vi "Template Rename.vi"(6 "ROI":string, 7 "Root Path":path, 8 "error in (no error)":errorcluster, 9 "Project List Idx":u16, 10 "Project List":string[](array[string])) -> (0 "error out":errorcluster)   [LabVIEW 2019]
uses:
  ROI/Controls/ROI_List_Action.ctl
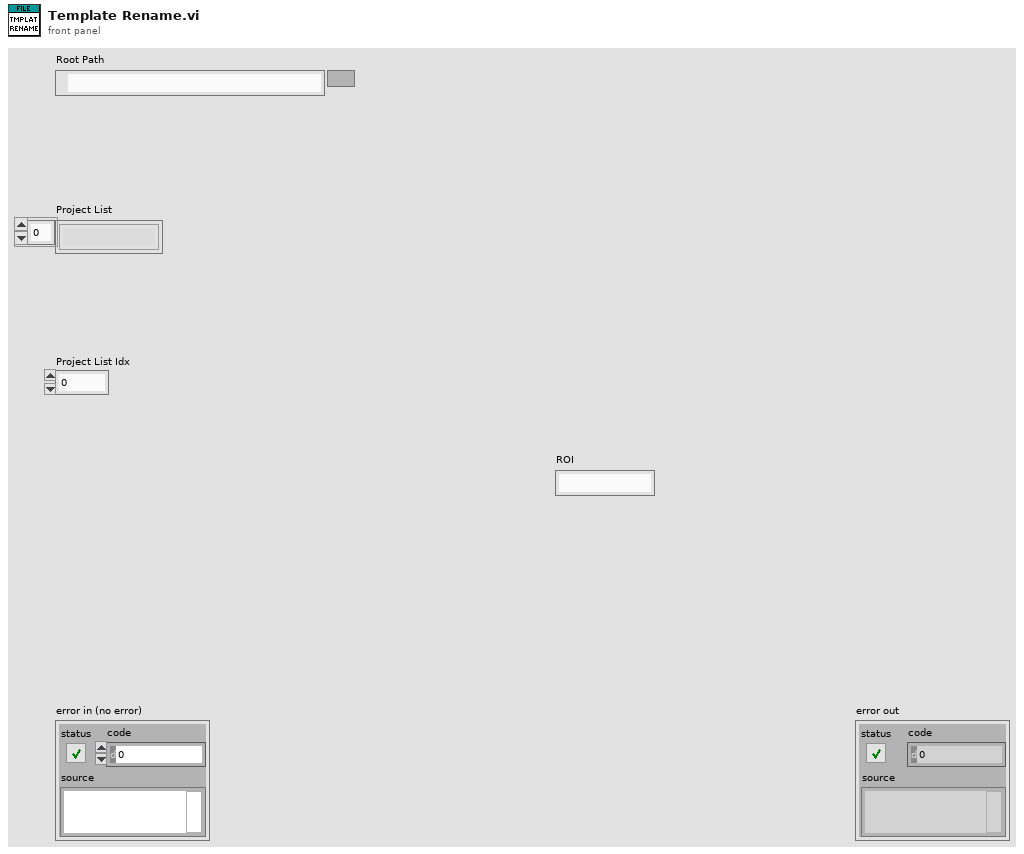
[diagram p1: front panel]
types:
  T1 = typedef "ROI_List_Action.ctl" = enum16{"Init", "Add ROI", "Delete ROI", "Get All ROI", "Get Specific ROI", "Set Analysis Setting", "Set Process Setting", "Replace All Entries", "ROIEntryBackup", "ROIEntryBackupClear", "ROIEntryReturn"}
  T2 = typedef "Vision_DataEntry.ctl" = cluster{"vROIName":string, "vROIContour":cluster{"Contour Type":u32, "ROI Type":u32, "Points":i32[]}, "ProcessSetting":T3[], "Analysis_Setting":T5}
  T3 = typedef "Process_Setting.ctl" = cluster{"Enum_PreProcess":T4, "Parameter":string}
  T4 = typedef "VisionProcessName.ctl" = enum16{"*CamParameter*", "CamAttributes", "*Preprocess*", "CG_Brightness", "C_Plane Extraction", "C_Threshold", "G_Lookup Table", "G_Threshold"}
  T5 = typedef "Analysis_Setting.ctl" = cluster{"PreProcess":T6, "Parameter":string}
  T6 = typedef "V_Analysis_Type.ctl" = enum16{"None", "C_Color Pattern Matching", "G_PatternMatching", "G_ShapeDectect", "G_GeometricMatch", "B_Area Check"}
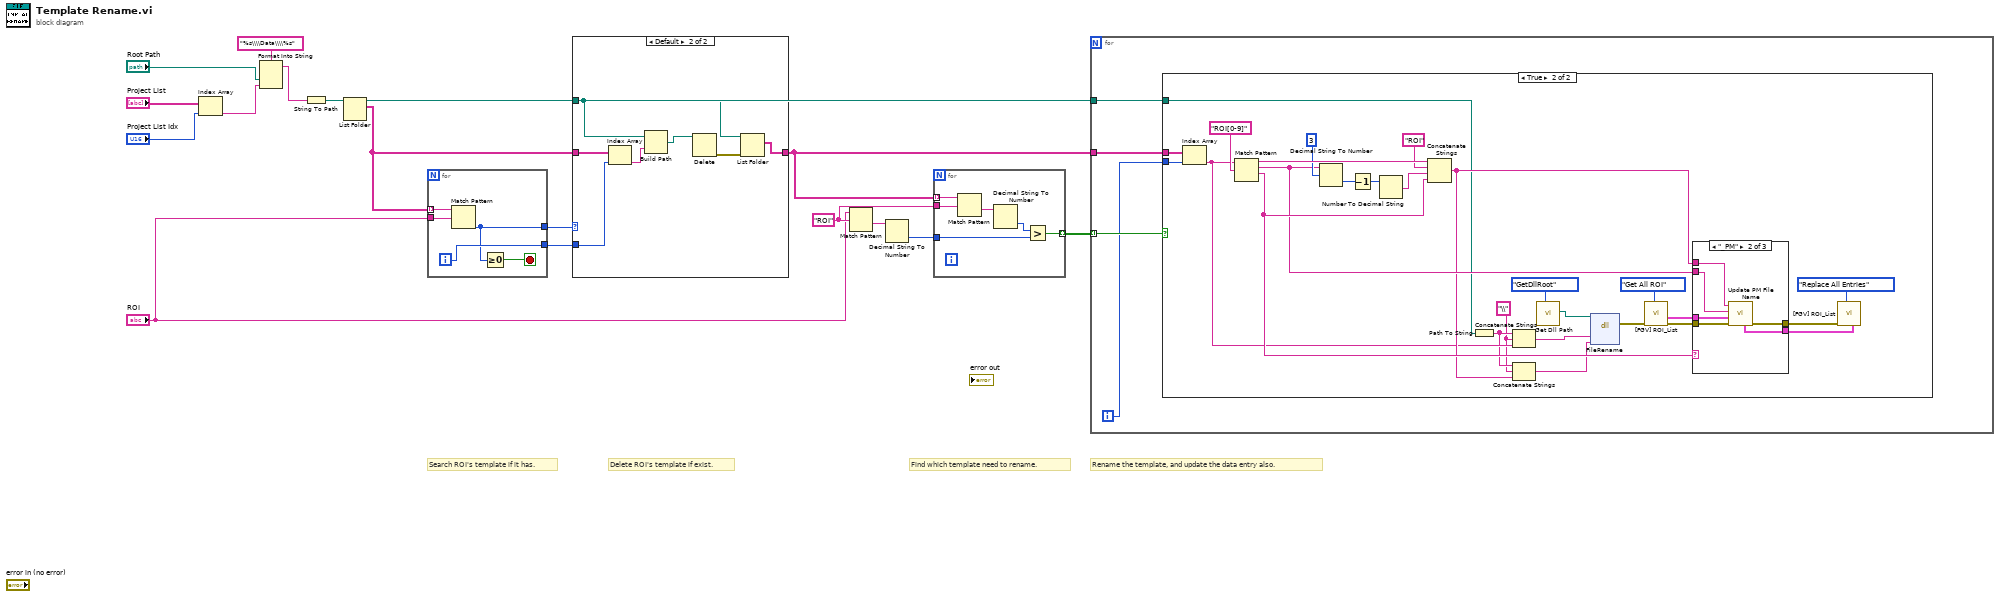
[diagram p0: block diagram]
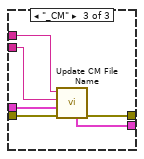
[diagram p4: hidden frame]
diagram:
  w17 = "ROI" ("regular expression")
  # "Rename the template, and update the data entry also."
  # "Find which template need to rename."
  # "Delete ROI's template if exist."
  # "Search ROI's template if it has."
  n1 = Index Array(array="Project List", index="Project List Idx") -> (element=w5:string)
  n2 = Format Into String(format string="%s\\\\Data\\\\%s", "Root Path", w5) -> (resulting string=w4:string)  [unwired: 2 in, 1 out]
  n3 = String To Path(string=w4) -> (path=w3:path)
  n4 = List Folder(path=w3) -> (path out=w10:path, filenames=w1:string[])  [unwired: 3 in, 2 out]
  n5 = for {
    tunnel: w1 -> [w22] mode=indexing
    tunnel: [w19] -> w16
    tunnel: [w21] -> w15
    tunnel: "ROI" -> [w18]
    i -> [w21]
    stop <- w20 stop-if-true
    n6 = Match Pattern(string=w22, regular expression=w18) -> (offset past match=w19:i32)  [unwired: 1 in, 3 out]
    n7 = Greater Or Equal To 0?(x=w19) -> (x >= 0?=w20:bool)
  }
  n8 = case shown="Default" w16 {
    tunnel: w1 -> [w23 w29]
    tunnel: w15 -> [_ w30]
    tunnel: [w23 w27] -> w9
    tunnel: w10 -> [_ w28]
    frame -1 {
    }
    frame Default {
      n9 = Index Array(array=w29, index=w30) -> (element=w26:string)
      n10 = Build Path(base path=w28, name or relative path=w26) -> (appended path=w25:path)
      n11 = Delete(path (use dialog)=w25) -> (error out=w24:errorcluster)  [unwired: 4 in, 2 out]
      n12 = List Folder(path=w28, error in=w24) -> (filenames=w27:string[])  [unwired: 2 in, 3 out]
    }
  }
  n13 = Match Pattern(string="ROI", regular expression=w17) -> (after substring=w12:string)  [unwired: 1 in, 3 out]
  n14 = Decimal String To Number(string=w12) -> (number=w11:i32)  [unwired: 2 in, 1 out]
  n15 = for {
    tunnel: w9 -> [w36] mode=indexing
    tunnel: [w33] -> w13 mode=indexing
    tunnel: w17 -> [w32]
    tunnel: w11 -> [w31]
    n16 = Match Pattern(string=w36, regular expression=w32) -> (after substring=w35:string)  [unwired: 1 in, 3 out]
    n17 = Decimal String To Number(string=w35) -> (number=w34:i32)  [unwired: 2 in, 1 out]
    n18 = Greater?(x=w34, y=w31) -> (0:w33:bool)
  }
  n19 = for {
    tunnel: w13 -> [w40] mode=indexing
    tunnel: w10 -> [w39]
    tunnel: w9 -> [w38]
    i -> [w37]
    n20 = case shown="True" w40 {
      tunnel: w38 -> [_ w54]
      tunnel: w37 -> [_ w62]
      tunnel: w39 -> [_ w56]
      frame False {
      }
      frame True {
        w41 = "\\"
        n21 = Index Array(array=w54, index=w62) -> (element=w55:string)
        n22 = Match Pattern(string=w55, regular expression="ROI[0-9]") -> (before substring=w64:string, match substring=w58:string, after substring=w59:string)  [unwired: 1 in, 1 out]
        n23 = Decimal String To Number(string=w58, offset=3) -> (number=w65:i32)  [unwired: 1 in, 1 out]
        n24 = Decrement(x=w65) -> (x-1=w66:i32)
        n25 = Number To Decimal String(number=w66) -> (decimal integer string=w63:string)  [unwired: 1 in]
        n26 = Concatenate Strings(w64, "ROI" ("string"), w63, w59) -> (w57:string)
        n27 = Path To String(path=w56) -> (string=w43:string)
        n28 = Concatenate Strings(w43, w41, w55) -> (w44:string)
        n29 = Concatenate Strings(w43, w41, w57) -> (w42:string)
        n30 = call "Get Dll Path.vi"("Action"=enum16{"WriteDllRoot", "GetDllRoot"}."GetDllRoot") -> ("Dll Root Path"=w45:path)  [unwired: 10 in]
        n31 = dll-call lib="C:/Users/user/Desktop/Smasoft/Project/iVision/20161003 Auto ROI/iVision_20161007_V1.6-3/SubVIs/File Name Dll/File Rename DLL.dll" fn="FileRename"(path in=w45, "OldName"=w44, "NewName"=w42) -> (error out=w47:errorcluster)  [unwired: 5 in, 1 out]
        n32 = call "[FGV] ROI_List.vi"("Action"=ROI_List_Action."Get All ROI", "error in (no error)"=w47) -> ("error out"=w52:errorcluster, "All ROI"=w48:T2[])  [unwired: 7 in, 1 out]
        n33 = case shown="\"_PM\"" w59 {
          tunnel: w52 -> [w69 w75 w81]
          tunnel: [w69 w74 w78] -> w50
          tunnel: [w68 w73 w79] -> w49
          tunnel: w48 -> [w68 w72 w80]
          tunnel: w58 -> [_ w70 w77]
          tunnel: w57 -> [_ w71 w76]
          frame Default {
          }
          frame "_PM" {
            n34 = call "Update PM File Name.vi"("error in (no error)"=w75, "All ROI In"=w72, "Old ROI Name"=w70, "New Template Name"=w71) -> ("error out"=w74:errorcluster, "All ROI Out"=w73:T2[])  [unwired: 6 in]
          }
          frame "_CM" {
            n35 = call "Update CM File Name.vi"("error in (no error)"=w81, "All ROI In"=w80, "Old ROI Name"=w77, "New Template Name"=w76) -> ("error out"=w78:errorcluster, "All ROI Out"=w79:T2[])  [unwired: 6 in]
          }
        }
        n36 = call "[FGV] ROI_List.vi"("ROIEntriesIn"=w49, "Action"=ROI_List_Action."Replace All Entries", "error in (no error)"=w50) -> ()  [unwired: 6 in, 3 out]
      }
    }
  }
